vi "CopilotControls.vi"() -> ()   [LabVIEW 2019]
uses:
  <vilib>/Rock Robotics/WPI/ThirdParty/Phoenix-LabVIEW/Motor Controller/Controls/CTRE_Phoenix_MotorControl_ControlMode.ctl
  Driver Globals.vi
panel:
  in  "Derivative":dbl
  in  "Integral":dbl
  in  "Proportional":dbl
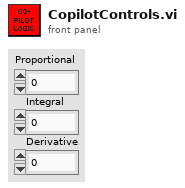
[diagram p1: front panel]
types:
  T1 = enum16{"DemandType_Neutral", "DemandType_AuxPID", "DemandType_ArbitraryFeedForward"}
  T2 = typedef "CTRE_Phoenix_MotorControl_ControlMode.ctl" = u16
  T3 = typedef "Color Sensor V3 DevRef.ctl" = cluster{"I2CDevRef":T4}
  T4 = typedef "WPI_I2CDevRef.ctl" = cluster{"DevStatus":errorcluster, "Device Address":u8, "Handle":i32, "I2C Bus":T5}
  T5 = typedef "i2c_bus.ctl" = enum16{"I2C On-Board", "I2C MXP", "Invalid"}
  T6 = typedef "WPI_MotorControlDeviceRef.ctl" = cluster{"DeviceStatus":errorcluster, "Type":T7, "PWM":cluster{"PWM Channel":T8, "DeadBand":T9}, "CAN":cluster{"Device Number":u8, "SetOutput VI Ref":variant, "GetOutput VI Ref":variant, "Enable VI Ref":variant, "Disable VI Ref":variant, "Data":variant}, "Invert":bool, "DIO PWM":cluster{"PWM \"Enable\" Channel":T8, "DIOChannel":T10, "PWM Rate":dbl}}
  T7 = typedef "WPI_MotorControlType.ctl" = enum16{"PWM", "CAN", "DIO PWM"}
  T8 = typedef "FPGA_DIOPWMChannel.ctl" = enum8{"PWM 0", "PWM 1", "PWM 2", "PWM 3", "PWM 4", "PWM 5", "PWM 6", "PWM 7", "PWM 8", "PWM 9", "PWM MXP 0", "PWM MXP 1", "PWM MXP 2", "PWM MXP 3", "PWM MXP 4", "PWM MXP 5", "PWM MXP 6", "PWM MXP 7", "PWM MXP 8", "PWM MXP 9", "Invalid"}
  T9 = typedef "WPI_PWMDeadband.ctl" = cluster{"Name":string, "maxPositivePwm":i32, "minPositivePwm":i32, "centerPwm":i32, "maxNegativePwm":i32, "minNegativePwm":i32, "angularRange":u16}
  T10 = typedef "FPGA_DIOChannel.ctl" = enum8{"DIO 0", "DIO 1", "DIO 2", "DIO 3", "DIO 4", "DIO 5", "DIO 6", "DIO 7", "DIO 8", "DIO 9", "DIO MXP 0", "DIO MXP 1", "DIO MXP 2", "DIO MXP 3", "DIO MXP 4", "DIO MXP 5", "DIO MXP 6", "DIO MXP 7", "DIO MXP 8", "DIO MXP 9", "DIO MXP 10", "DIO MXP 11", "DIO MXP 12", "DIO MXP 13", "DIO MXP 14", "DIO MXP 15", "SPI Port CS1", "SPI Port CS2", "SPI Port CS3", "SPI Port MISO", "SPI Port MOSI", "Invalid"}
  T11 = typedef "WPI_EncoderDevRef.ctl" = cluster{"DevStatus":errorcluster, "EncoderIndex":T12, "CounterIndex":T13, "DistancePerCount":dbl, "Decoding Type":T14}
  T12 = typedef "FPGA_EncoderIdx.ctl" = enum8{"Enc 0", "Enc 1", "Enc 2", "Enc 3", "Enc 4", "Enc 5", "Enc 6", "Enc 7", "Invalid"}
  T13 = typedef "FPGA_CounterCtrSystemIndex.ctl" = enum8{"Ctr 0", "Ctr 1", "Ctr 2", "Ctr 3", "Ctr 4", "Ctr 5", "Ctr 6", "Ctr 7", "Invalid"}
  T14 = typedef "WPI_EncoderType.ctl" = enum16{"1x", "2x", "4x"}
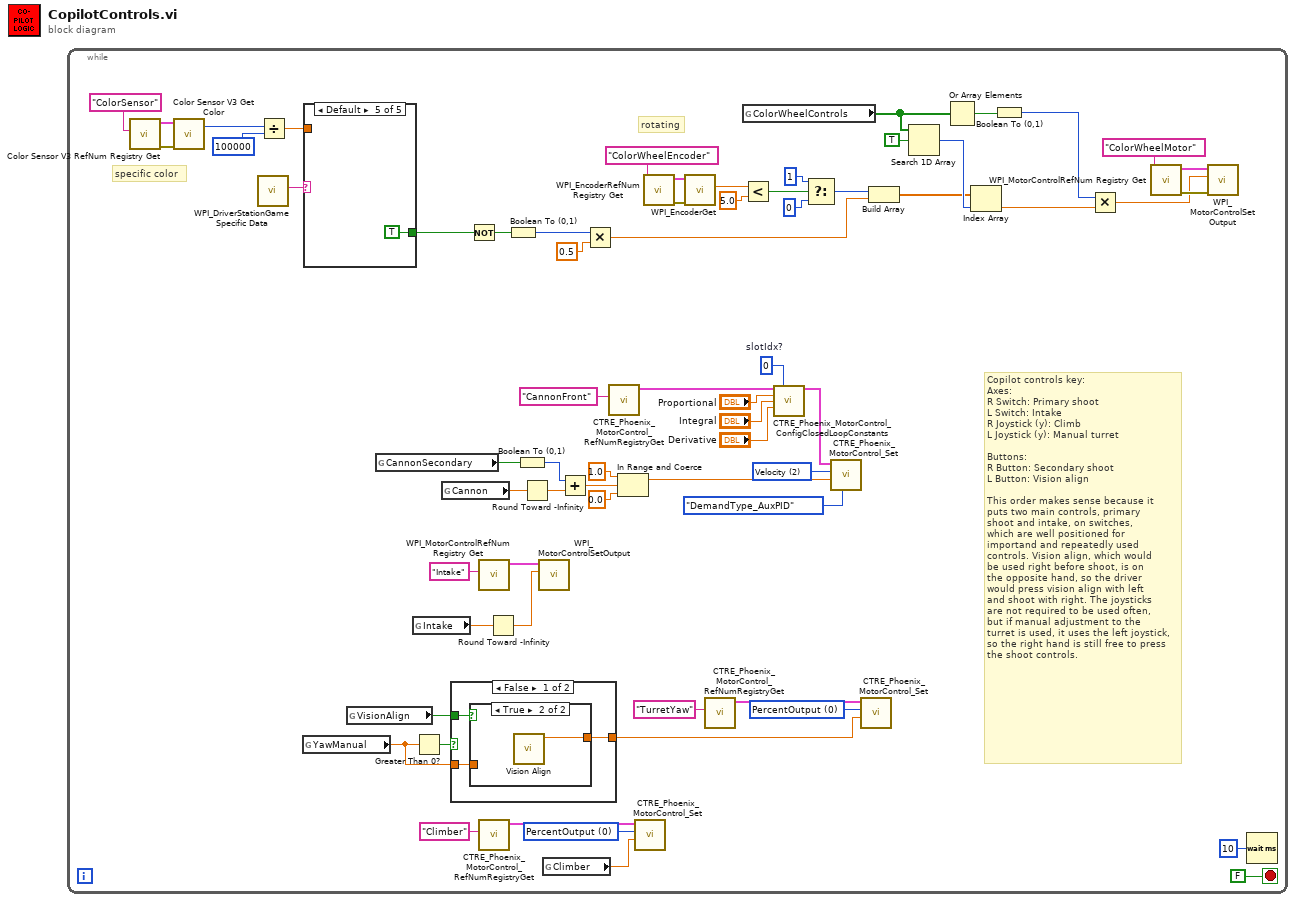
[diagram p0: block diagram]
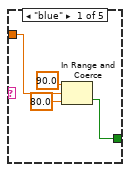
[diagram p4: hidden frame]
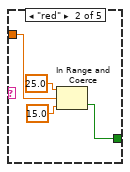
[diagram p5: hidden frame]
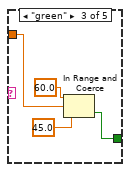
[diagram p6: hidden frame]
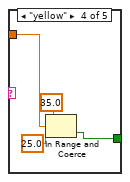
[diagram p7: hidden frame]
diagram:
  n1 = while {
    stop <- FALSE stop-if-true
    w16 = T2 0 items=["PercentOutput"=0, "Position"=1, "Velocity"=2, "Current"=3, "Follower"=5, "MotionProfile"=6, "MotionMagic"=7, "MotionProfileArc"=10, "Disabled"=15] ("Control Mode")
    w19 = T2 0 items=["PercentOutput"=0, "Position"=1, "Velocity"=2, "Current"=3, "Follower"=5, "MotionProfile"=6, "MotionMagic"=7, "MotionProfileArc"=10, "Disabled"=15] ("Control Mode")
    w23 = 0  # slotIdx?
    w26 = T2 2 items=["PercentOutput"=0, "Position"=1, "Velocity"=2, "Current"=3, "Follower"=5, "MotionProfile"=6, "MotionMagic"=7, "MotionProfileArc"=10, "Disabled"=15] ("Control Mode")
    # "Copilot controls key:\nAxes:\nR Switch: Primary shoot\nL Switch: Intake\nR Joystick (y): Climb\nL Joystick (y): Manual turret\n\nButtons:\nR Button: Secondary shoot\nL Button: Vision align\n\nThis order makes sense because it\nputs two main controls, primary\nshoot and intake, on switches,\nwhich are well positioned for\nimportand and repeatedly used\ncontrols. Vision align, which would\nbe used right before shoot, is on\nthe opposite hand, so the driver\nwould press vision align with left\nand shoot with right. The joysticks\nare not required to be used often,\nbut if manual adjustment to the\nturret is used, it uses the left joystick,\nso the right hand is still free to press\nthe shoot controls."
    # "specific color"
    # "rotating"
    n2 = call <vilib>:"Color Sensor V3 RefNum Registry Get.vi"("refnum name"="ColorSensor") -> ("error out"=w61:errorcluster, "ColorSensorDevRef"=w60:T3)  [unwired: 9 in]
    n3 = call <vilib>:"Color Sensor V3 Get Color.vi"("error in (no error)"=w61, "ColorSensorDevRef"=w60) -> ("Color"=w58:u32)  [unwired: 6 in, 3 out]
    n4 = call <vilib>:"WPI_DriverStationGame Specific Data.vi"() -> ("Game Specific Data"=w62:string)  [unwired: 11 in]
    n5 = Divide(x=w58, y=u32 100000) -> (x/y=w56:dbl)
    n6 = global read "Driver Globals.vi" "YawManual"() -> (w10:dbl)
    n7 = case shown="Default" w62 {
      tunnel: w56 -> [w76 w80 w84 w88 _]
      tunnel: [w73 w77 w81 w85 TRUE] -> w1
      frame "blue" {
        n8 = In Range and Coerce(upper limit=90.0, x=w76, lower limit=80.0) -> (In Range?=w73:bool)  [unwired: 1 out]
      }
      frame "red" {
        n9 = In Range and Coerce(upper limit=25.0, x=w80, lower limit=15.0) -> (In Range?=w77:bool)  [unwired: 1 out]
      }
      frame "green" {
        n10 = In Range and Coerce(upper limit=60.0, x=w84, lower limit=45.0) -> (In Range?=w81:bool)  [unwired: 1 out]
      }
      frame "yellow" {
        n11 = In Range and Coerce(upper limit=35.0, x=w88, lower limit=25.0) -> (In Range?=w85:bool)  [unwired: 1 out]
      }
      frame Default {
      }
    }
    n12 = global read "Driver Globals.vi" "VisionAlign"() -> (w12:bool)
    n13 = global read "Driver Globals.vi" "CannonSecondary"() -> (w13:bool)
    n14 = global read "Driver Globals.vi" "Intake"() -> (w4:dbl)
    n15 = Greater Than 0?(x=w10) -> (x > 0?=w18:bool)
    n16 = global read "Driver Globals.vi" "Cannon"() -> (w11:dbl)
    n17 = case shown="False" w18 {
      tunnel: w12 -> [w69 _]
      tunnel: [w67 w72] -> w14
      tunnel: w10 -> [w68 w72]
      frame False {
        n18 = case shown="True" w69 {
          tunnel: w68 -> [w70 _]
          tunnel: [w70 w71] -> w67
          frame False {
          }
          frame True {
            n19 = call "Vision Align.vi"() -> ("YawOut"=w71:dbl)  [unwired: 11 in]
          }
        }
      }
      frame True {
      }
    }
    n20 = Not(x=w1) -> (.not. x?=w2:bool)
    n21 = call <vilib>:"WPI_MotorControlRefNum Registry Get.vi"("refnum name"="Intake") -> ("MotorControlDevRef"=w33:T6)  [unwired: 9 in, 1 out]
    n22 = call <vilib>:"CTRE_Phoenix_MotorControl_RefNumRegistryGet.vi"("refnum name"="Climber") -> ("PhoenixMotorControlDevRef"=w20:T6)  [unwired: 9 in, 1 out]
    n23 = Round Toward -Infinity(1:w4) -> (0:w22:dbl)
    n24 = Boolean To (0,1)(Boolean=w2) -> (0, 1=w3:i16)
    n25 = Boolean To (0,1)(Boolean=w13) -> (0, 1=w24:i16)
    n26 = Round Toward -Infinity(1:w11) -> (0:w25:dbl)
    n27 = call <vilib>:"WPI_MotorControlSetOutput.vi"("Output"=w22, "MotorControlDevRef"=w33) -> ()  [unwired: 7 in, 3 out]
    n28 = global read "Driver Globals.vi" "Climber"() -> (w9:dbl)
    n29 = Add(x=w24, y=w25) -> (x+y=w35:dbl)
    n30 = Multiply(x=w3, y=0.5) -> (x*y=w45:dbl)
    n31 = call <vilib>:"CTRE_Phoenix_MotorControl_RefNumRegistryGet.vi"("refnum name"="CannonFront") -> ("PhoenixMotorControlDevRef"=w32:T6)  [unwired: 9 in, 1 out]
    n32 = In Range and Coerce(upper limit=1.0, x=w35, lower limit=0.0) -> (coerced(x)=w38:dbl)  [unwired: 1 out]
    n33 = call <vilib>:"CTRE_Phoenix_MotorControl_Set.vi"("Output"=w9, "Control Mode"=w19, "PhoenixMotorControlDevRef"=w20) -> ()  [unwired: 7 in, 2 out]
    n34 = call <vilib>:"WPI_EncoderRefNum Registry Get.vi"("refnum name"="ColorWheelEncoder") -> ("error out"=w64:errorcluster, "EncoderDevRef"=w65:T11)  [unwired: 9 in]
    n35 = call <vilib>:"WPI_EncoderGet.vi"("error in (no error)"=w64, "EncoderDevRef"=w65) -> ("Distance"=w51:dbl)  [unwired: 4 in, 5 out]
    n36 = call <vilib>:"CTRE_Phoenix_MotorControl_RefNumRegistryGet.vi"("refnum name"="TurretYaw") -> ("PhoenixMotorControlDevRef"=w17:T6)  [unwired: 9 in, 1 out]
    n37 = global read "Driver Globals.vi" "ColorWheelControls"() -> (w8:bool[])
    n38 = Less?(x=w51, y=5.0) -> (x < y?=w49:bool)
    n39 = call <vilib>:"CTRE_Phoenix_MotorControl_ConfigClosedLoopConstants.vi"("PhoenixMotorControlDevRef"=w32, "slotIdx"=w23, "P"="Proportional", "I"="Integral", "D"="Derivative") -> ("PhoenixMotorControlDevRef"=w30:T6)  [unwired: 9 in, 1 out]
    n40 = Select(t=i16 1, s=w49, f=i16 0) -> (s? t:f=w46:i16)
    n41 = call <vilib>:"CTRE_Phoenix_MotorControl_Set.vi"("DemandType"=T1."DemandType_AuxPID", "Output"=w38, "Control Mode"=w26, "PhoenixMotorControlDevRef"=w30) -> ()  [unwired: 6 in, 2 out]
    n42 = call <vilib>:"CTRE_Phoenix_MotorControl_Set.vi"("Output"=w14, "Control Mode"=w16, "PhoenixMotorControlDevRef"=w17) -> ()  [unwired: 7 in, 2 out]
    n43 = Build Array(w46, w45) -> (w41:dbl[])
    n44 = Search 1D Array(1D array=w8, element=TRUE) -> (index of element=w42:i32)  [unwired: 1 in]
    n45 = Or Array Elements(Boolean array=w8) -> (logical OR=w44:bool)
    n46 = Index Array(array=w41, index=w42) -> (element=w6:dbl)
    n47 = Boolean To (0,1)(Boolean=w44) -> (0, 1=w5:i16)
    n48 = Multiply(x=w5, y=w6) -> (x*y=w40:dbl)
    n49 = call <vilib>:"WPI_MotorControlRefNum Registry Get.vi"("refnum name"="ColorWheelMotor") -> ("error out"=w53:errorcluster, "MotorControlDevRef"=w54:T6)  [unwired: 9 in]
    n50 = call <vilib>:"WPI_MotorControlSetOutput.vi"("error in (no error)"=w53, "Output"=w40, "MotorControlDevRef"=w54) -> ()  [unwired: 6 in, 3 out]
    n51 = Wait (ms)(milliseconds to wait=u32 10) -> ()  [unwired: 1 out]
  }
